vi "Global_HoodSensorPos.vi"() -> ()   [LabVIEW 2017]
panel:
  in  "Hood Sensor Position":dbl
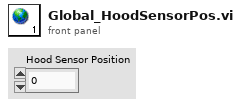
[diagram p1: front panel]
diagram:
